vi "Check Valid Move.vi"(8 "Vertex":cluster{"row":i32, "col":i32}, 9 "Parent":cluster{"row":i32, "col":i32}, 11 "Map in":T1(c390)) -> (2 "Valid Move?":bool, 3 "Map out":T1(c390))   [LabVIEW 2021, in "d12.lvlib"]
uses:
  d12.lvlib
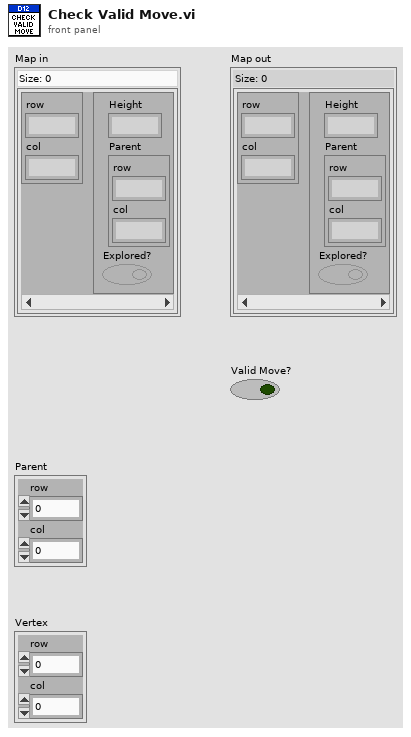
[diagram p1: front panel]
types:
  T1 = map{cluster{"row":i32, "col":i32}, cluster{"Height":i16, "Parent":cluster{"row":i32, "col":i32}, "Explored?":bool}}
  T2 = cluster{"Height":i16, "Parent":cluster{"row":i32, "col":i32}, "Explored?":bool}
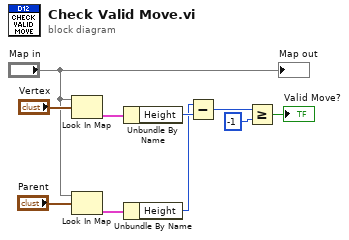
[diagram p0: block diagram]
diagram:
  n1 = Look In Map(map="Map in", key="Vertex") -> (value=w10:T2)  [unwired: 1 in, 1 out]
  n2 = Look In Map(map="Map in", key="Parent") -> (value=w7:T2)  [unwired: 1 in, 1 out]
  n3 = Unbundle By Name(w10) -> ("Height"=w2:i16)
  n4 = Unbundle By Name(w7) -> ("Height"=w1:i16)
  n5 = Subtract(x=w1, y=w2) -> (x-y=w3:i16)
  n6 = Greater Or Equal?(x=w3, y=i16 -1) -> (x >= y?=→"Valid Move?":bool)
  "Map out" <- "Map in"
